vi "SLM_control_event_structure_example.vi"() -> ()   [LabVIEW 2023]
panel:
  in  "Grating Sliders":cluster{"Y":sgl, "X":sgl} {"X" min=0 max=10 step=0.01 scale=0.0..10.0; "Y" min=0 max=10 step=0.01 scale=0.0..10.0}
  in  "Megapixels y":i32=5
  in  "Megapixels x":i32=5
  in  "Phase Array":dbl[][](array[numeric])
  in  "Start/Stop":bool
  out "Phase Array Graph":dbl[][](graph)
  # "X"
  # "Y"
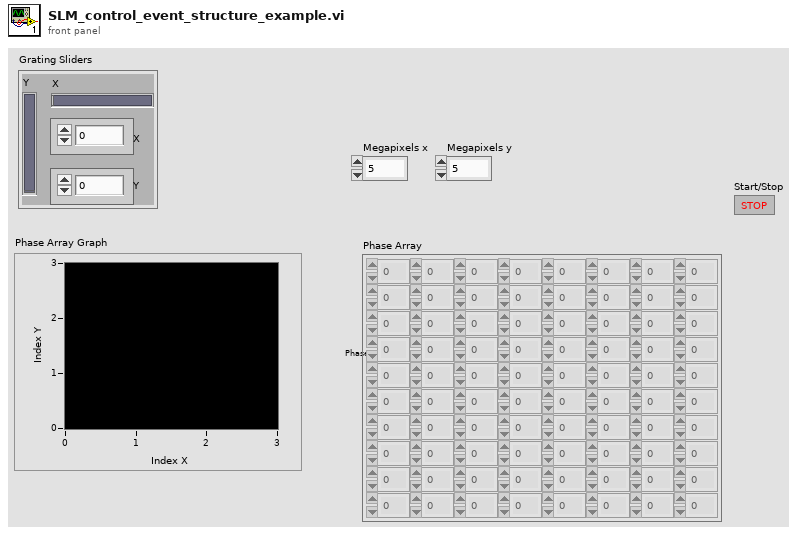
[diagram p1: front panel]
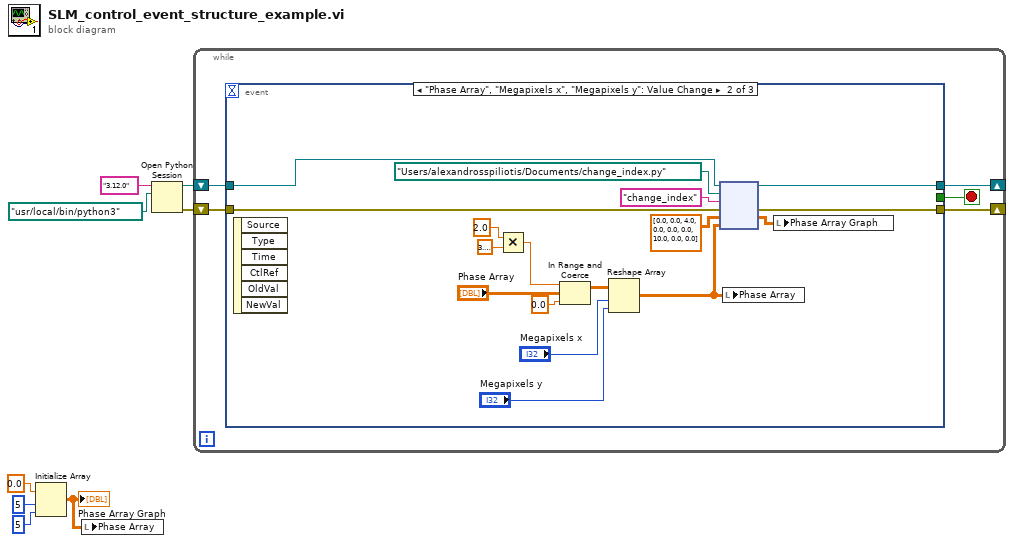
[diagram p0: block diagram]
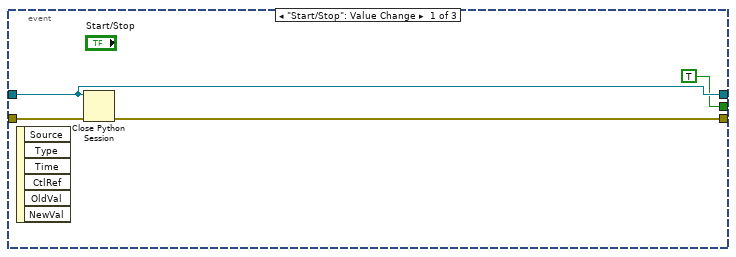
[diagram p2: hidden frame]
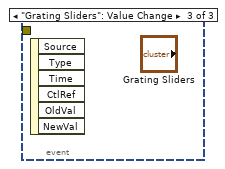
[diagram p3: hidden frame]
diagram:
  n1 = Initialize Array(0.0 ("element"), 5 ("dimension size"), 5 ("dimension size")) -> (w1:dbl[][])
  "Phase Array Graph" <- w1
  n2 = local write "Phase Array"(w1) -> ()
  n3 = Open Python Session(python version="3.12.0" ("Python version"), python path=path "/usr/local/bin/python3" ("Python path")) -> (session out=w8:refnum<k35>, error out=w7:errorcluster)  [unwired: 1 in]
  n4 = while {
    shift-right: [w10] -> _
    shift-left: w8 -> [w13]
    shift-right: [w11] -> _
    shift-left: w7 -> [w12]
    stop <- w9 stop-if-true
    n5 = event shown="[1] \"Phase Array\", \"Megapixels x\", \"Megapixels y\": Value Change" {
      selector: _ -> [_ _ _]
      dyn-events: _ -> [_ _ _]
      timeout: _ -> [_ _ _]
      tunnel: w13 -> [w15 w26 _]
      tunnel: w12 -> [w17 w24 _]
      tunnel: [w16 w23 _] -> w11
      tunnel: [w15 w25 _] -> w10
      tunnel: [TRUE ("Start/Stop") _ _] -> w9
      event "Start/Stop": Value Change {
        n6 = event-data() -> ()  [unwired: 1 in, 6 out]
        n7 = Close Python Session(session in=w15, error in=w17) -> (11:w16:errorcluster)
      }
      event "Phase Array", "Megapixels x", "Megapixels y": Value Change {
        n8 = event-data() -> ()  [unwired: 1 in, 6 out]
        n9 = Multiply(x=2.0, y=3.141592653589793) -> (x*y=w30:dbl)
        n10 = In Range and Coerce(upper limit=w30, x="Phase Array", lower limit=0.0) -> (coerced(x)=w31:dbl[][])  [unwired: 1 out]
        n11 = Reshape Array "Reshape Array"(w31, "Megapixels x", "Megapixels y") -> (w18:dbl[][])
        n12 = node(w26, path "/Users/alexandrosspiliotis/Documents/change_index.py" ("module path"), "change_index" ("function name"), w24, dbl[][] [[0.0, 0.0, 4.0], [0.0, 0.0, 0.0], [10.0, 0.0, 0.0]] ("Python Graph"), w18) -> (w25:refnum<k35>, w23:errorcluster, w19:dbl[][])  [unwired: 1 in, 2 out]
        n13 = local write "Phase Array"(w18) -> ()
        n14 = local write "Phase Array Graph"(w19) -> ()
      }
      event "Grating Sliders": Value Change {
        n15 = event-data() -> ()  [unwired: 1 in, 6 out]
      }
    }
  }
